vi "Auto Run.vi"() -> ()   [LabVIEW 2016]
uses:
  Ctls/Auto Steps.ctl
  <vilib>/vision/Image Controls.llb/IMAQ Image.ctl
  <vilib>/userdefined/High Color/IMAQdx.ctl
  <vilib>/vision/driver/IMAQdx.llb/IMAQdx Acquisition Mode.ctl
  LCOD.llb/GUI Command.ctl
  <vilib>/vision/driver/IMAQdx.llb/IMAQdx Buffer Number Mode.ctl
  <vilib>/Utility/config.llb/Read Key (Double).vi
  <vilib>/Utility/config.llb/Read Key (String).vi
  <vilib>/vision/driver/NI_Vision_Acquisition_Software.lvlib
  <vilib>/Utility/config.llb/NI_LVConfig.lvlib
panel:
  out "RobSnap":dbl[](array[numeric])
  out "RobRef":dbl[](array[numeric])
  out "CamRef":dbl[](array[numeric])
  out "Calibrate":string caption="值"
  out "Position":sgl[](array[numeric])
  out "Angle":sgl
  out "Top":cluster{"下边缘设置：":i32, "右边缘设置：":i32}
  out "Bottom":cluster{"上边缘设置：":i32, "右边缘设置：":i32}
  # "自动运行函数"
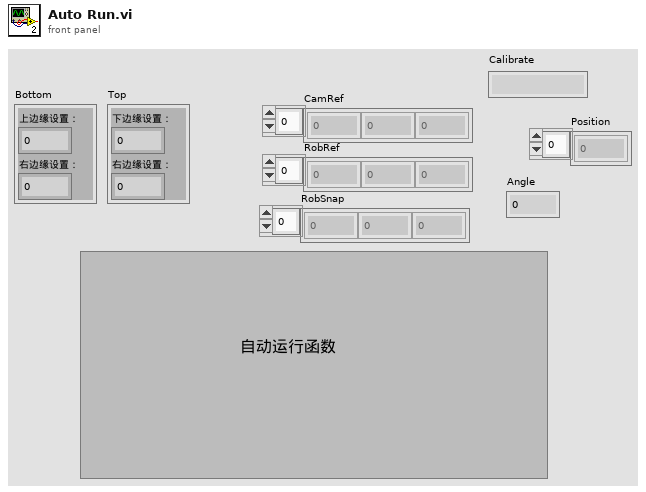
[diagram p1: front panel]
types:
  T1 = typedef "IMAQ Image.ctl" = refnum<image>
  T2 = typedef "Auto Steps.ctl" = enum16{"Nothing", "Initial", "ReadConf", "WaitTrigger", "SnapOnce", "Rotate180", "SnapSecond", "SendPos", "Error", "Pause", "Exit"}
  T3 = typedef "GUI Command.ctl" = enum16{"Under Range", "Get UI Setting", "错误代码处理", "保存数据", "保存图片", "Update Disp_Lists", "Update Sts", "Clear Disp_Lists", "Update Disp_Result", "Clear Disp_Result", "Set Passed Unit", "Set Failed Unit", "Set Total Unit", "Over Range"}
  T4 = typedef "NI_Vision_Acquisition_Software.lvlib/IMAQdx Acquisition Mode.ctl" = enum32{"One Shot", "Continuous"}
  T5 = typedef "IMAQdx.ctl" = refnum<k21>
  T6 = enum16{"Standard", "Buffered", "CRLF", "Immediate"}
  T7 = typedef "NI_Vision_Acquisition_Software.lvlib/IMAQdx Buffer Number Mode.ctl" = enum32{"Next", "Last", "Buffer Number", "Every", "Last New"}
  T8 = typedef "NI_LVConfig.lvlib/Config Data RefNum.ctl" = refnum<k1>
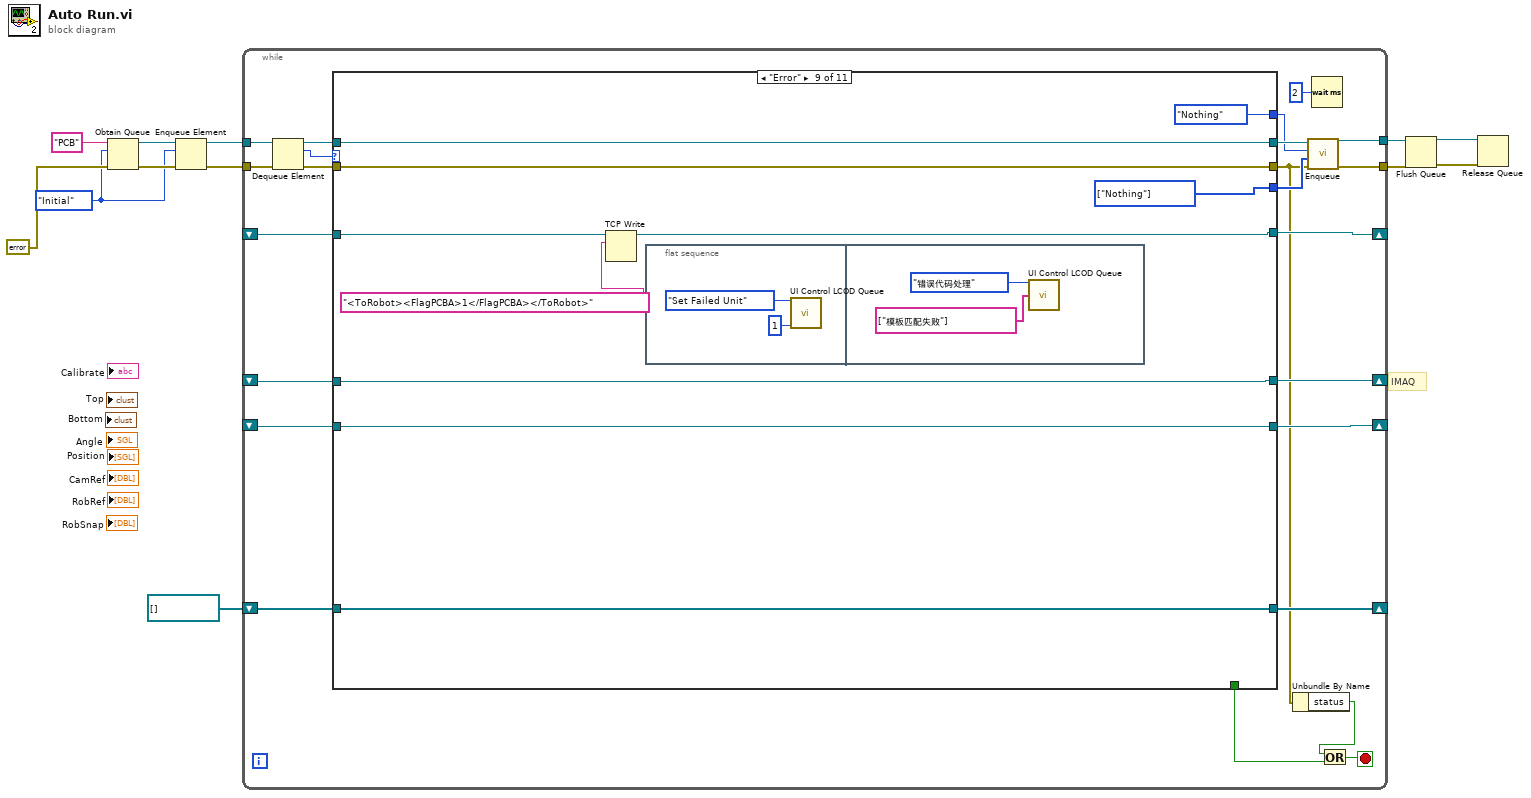
[diagram p0: block diagram]
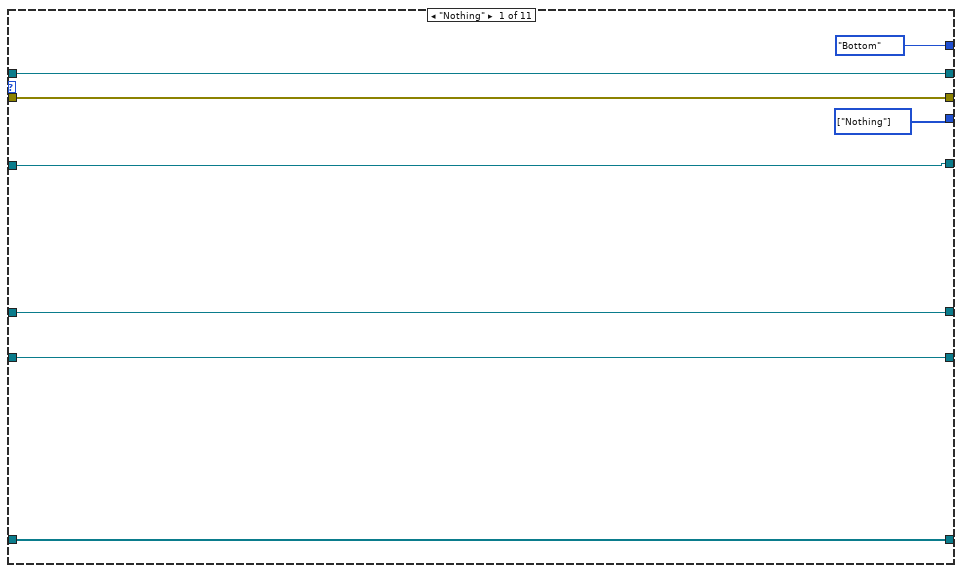
[diagram p2: hidden frame]
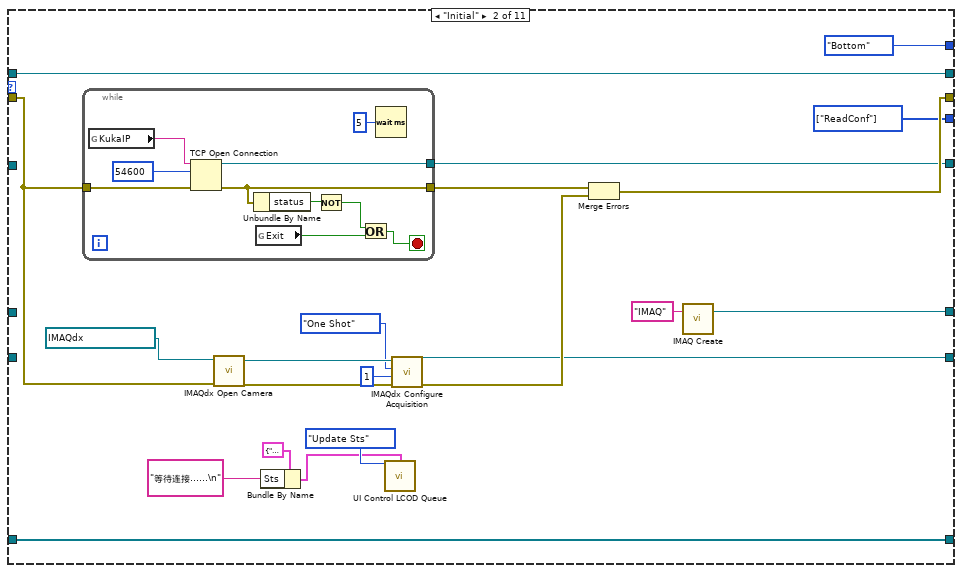
[diagram p3: hidden frame]
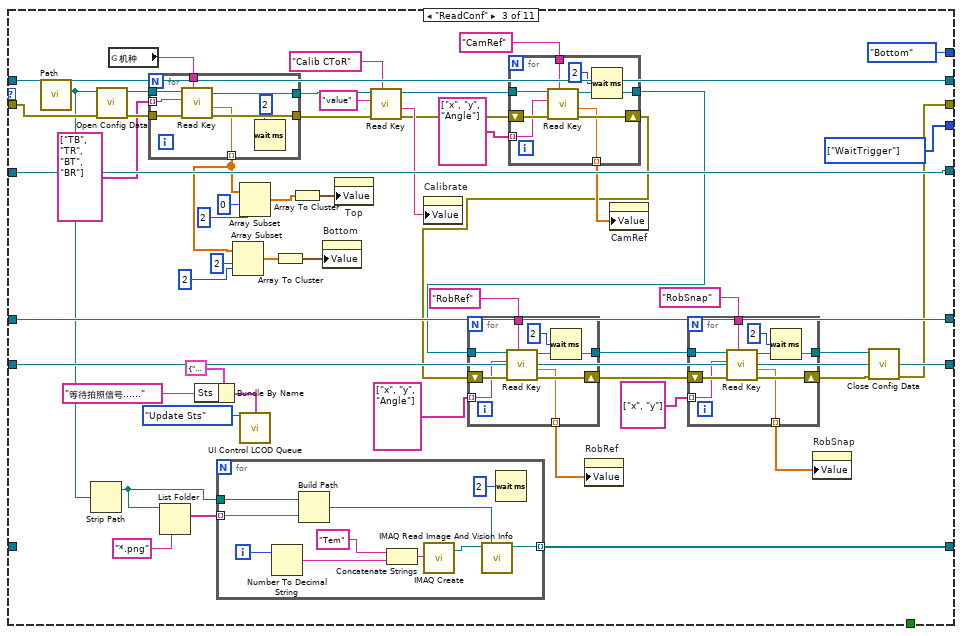
[diagram p4: hidden frame]
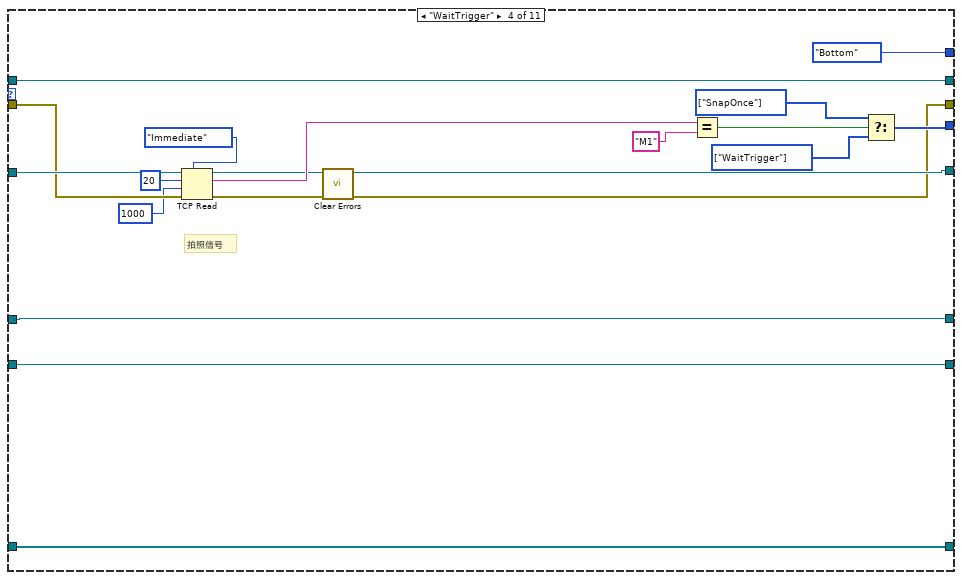
[diagram p5: hidden frame]
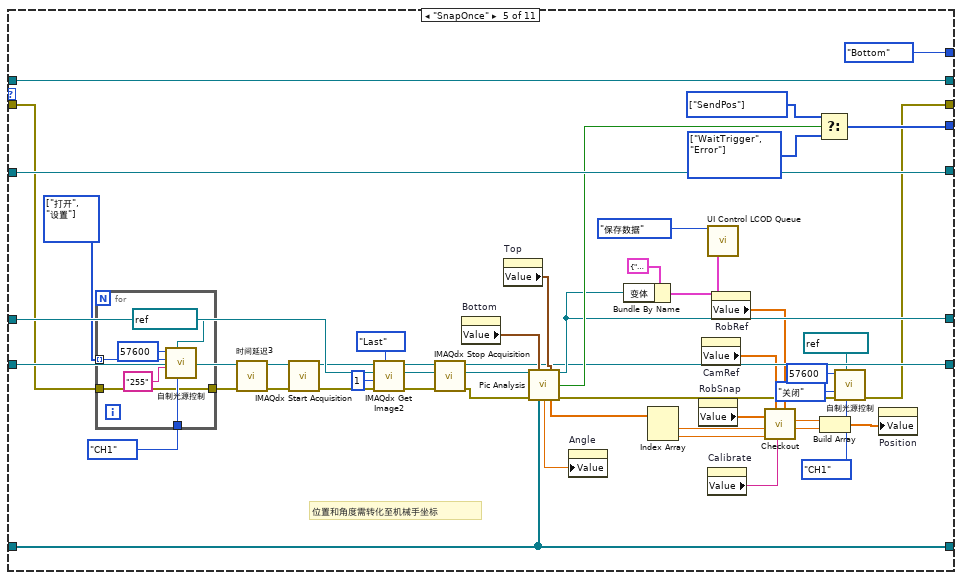
[diagram p6: hidden frame]
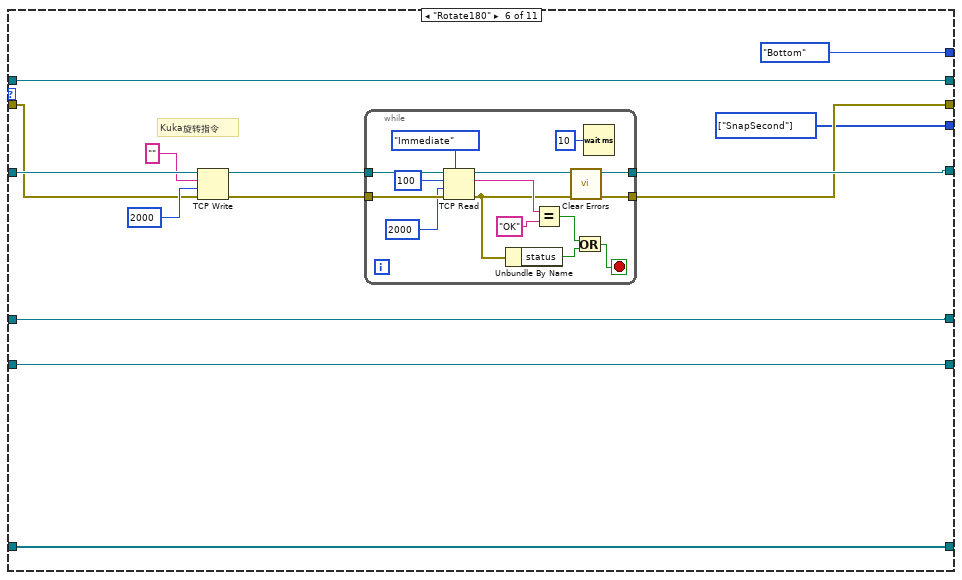
[diagram p7: hidden frame]
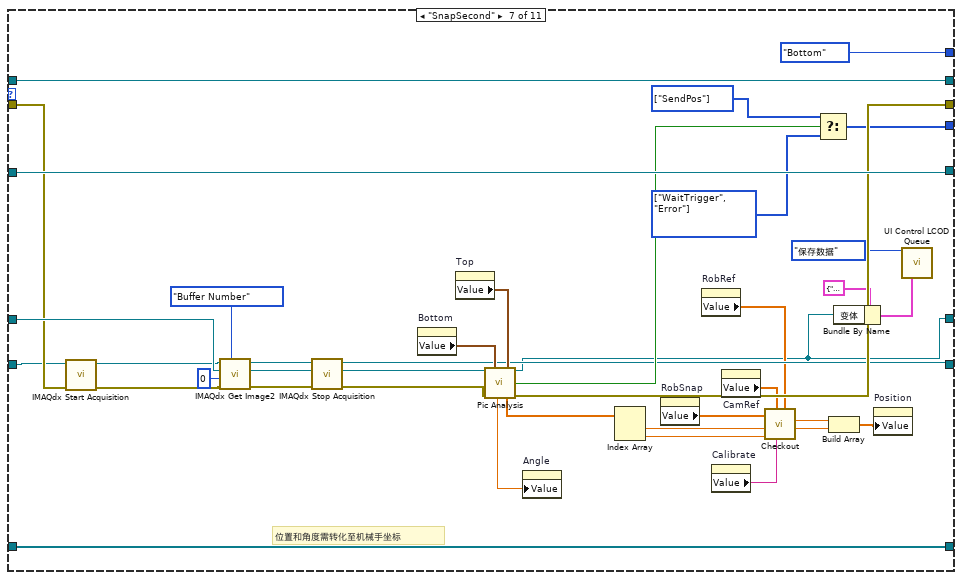
[diagram p8: hidden frame]
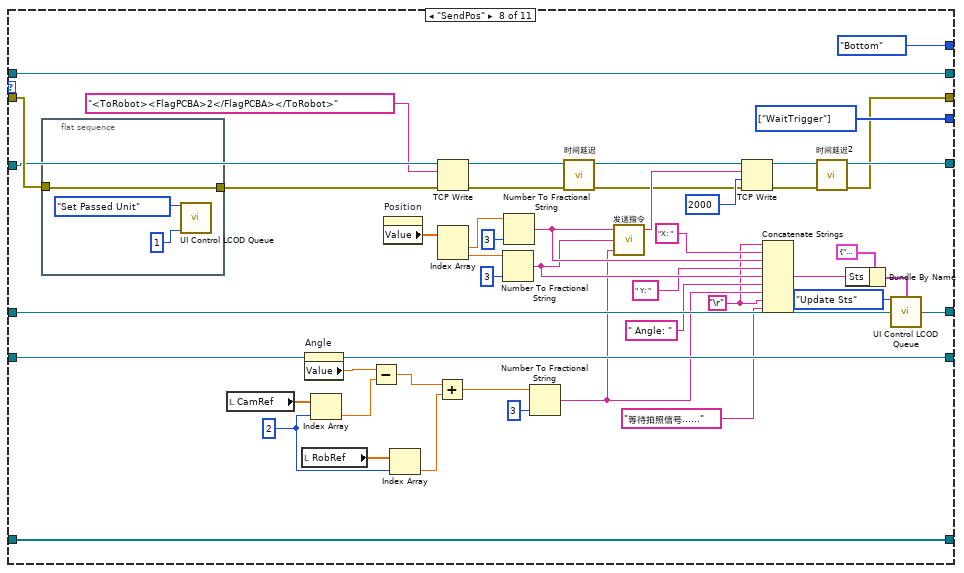
[diagram p9: hidden frame]
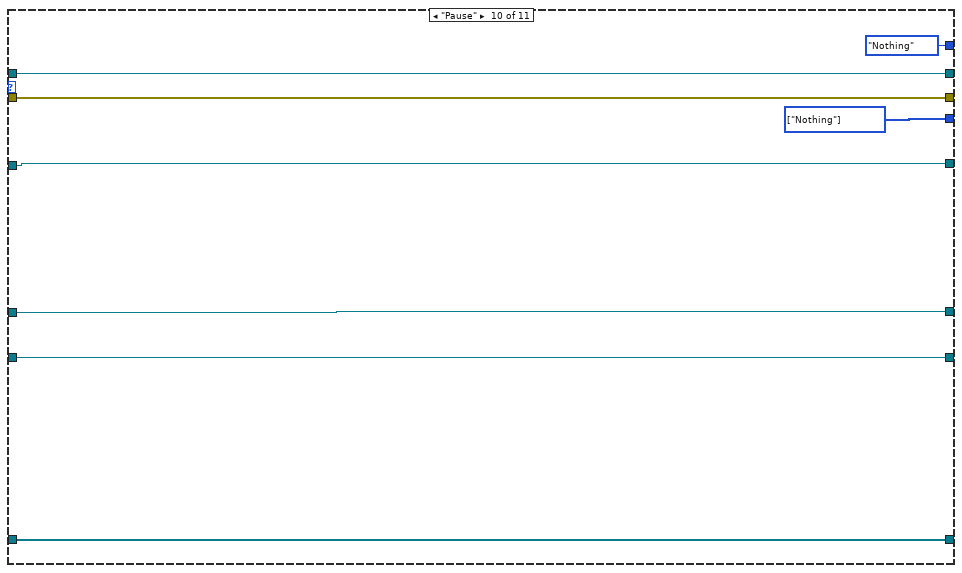
[diagram p10: hidden frame]
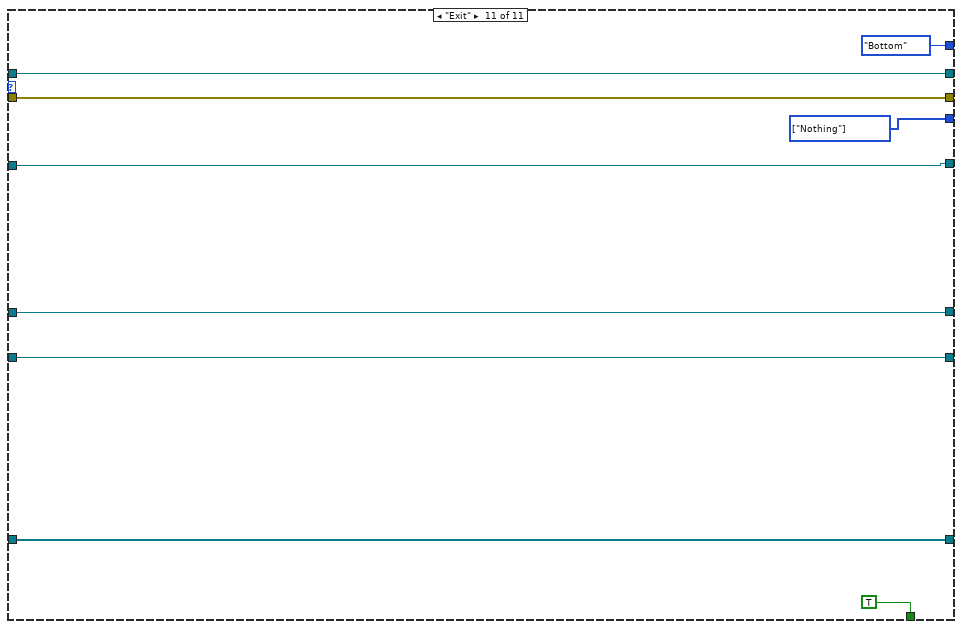
[diagram p11: hidden frame]
diagram:
  w8 = Auto_Steps."Initial"
  # "IMAQ"
  n1 = Obtain Queue(name (unnamed)="PCB" ("名称（未命名）"), element data type=w8, error in (no error)=errorcluster {"status"=FALSE, "code"=0, "source"=""} ("错误输入（无错误）")) -> (queue out=w10:refnum<queue>, error out=w9:errorcluster)  [unwired: 2 in, 1 out]
  n2 = Enqueue Element(queue=w10, element=w8, error in (no error)=w9) -> (queue out=w7:refnum<queue>, error out=w6:errorcluster)  [unwired: 1 in, 1 out]
  n3 = while {
    tunnel: w7 -> [w35]
    tunnel: w6 -> [w34]
    tunnel: [w29] -> w5
    tunnel: [w28] -> w4
    shift-right: [w24] -> _
    shift-left: _ -> [w22]
    shift-right: [w25] -> _
    shift-left: _ -> [w23]
    shift-right: [w21] -> _
    shift-left: _ -> [w20]
    shift-right: [w17] -> _
    shift-left: T1[] [] ("数组") -> [w18]
    stop <- w16 stop-if-true
    n4 = Dequeue Element(queue=w35, error in (no error)=w34) -> (queue out=w32:refnum<queue>, element=w33:T2, error out=w30:errorcluster)  [unwired: 1 in, 1 out]
    n5 = case shown="\"Error\"" w33 {
      tunnel: w32 -> [w43 w64 w126 w187 w234 w254 w306 w350 w363 w375 w383]
      tunnel: [w43 w64 w126 w187 w234 w254 w306 w350 w363 w375 w383] -> w31
      tunnel: w30 -> [w42 w58 w120 w183 w198 w250 w280 w320 w362 w374 w382]
      tunnel: [w42 w53 w118 w171 w193 w246 w297 w310 w362 w374 w382] -> w14
      tunnel: [w37 w51 w101 w179 w226 w242 w296 w331 w358 w369 w377] -> w19
      tunnel: [enum16{"Top", "Bottom", "Nothing"}."Bottom" ("Comd") enum16{"Top", "Bottom", "Nothing"}."Bottom" ("Comd") enum16{"Top", "Bottom", "Nothing"}."Bottom" ("Comd") enum16{"Top", "Bottom", "Nothing"}."Bottom" ("Comd") enum16{"Top", "Bottom", "Nothing"}."Bottom" ("Comd") enum16{"Top", "Bottom", "Nothing"}."Bottom" ("Comd") enum16{"Top", "Bottom", "Nothing"}."Bottom" ("Comd") enum16{"Top", "Bottom", "Nothing"}."Bottom" ("Comd") enum16{"Top", "Bottom", "Nothing"}."Nothing" ("Comd") enum16{"Top", "Bottom", "Nothing"}."Nothing" ("Comd") enum16{"Top", "Bottom", "Nothing"}."Bottom" ("Comd")] -> w26
      tunnel: [w38 w49 w123 w175 w205 w243 w281 w341 w359 w371 w378] -> w25
      tunnel: [w39 w54 w124 w176 w221 w244 w270 w342 w360 w372 w379] -> w24
      tunnel: w23 -> [w38 _ w123 w175 w208 w243 w278 w341 w359 w371 w378]
      tunnel: w22 -> [w39 _ w124 w176 w232 w244 w303 w342 w360 w372 w379]
      tunnel: [w40 w52 w125 w178 w233 w247 w304 w329 w356 w370 w380] -> w21
      tunnel: w20 -> [w40 _ w125 w186 w233 w252 w304 w319 w357 w370 w380]
      tunnel: [_ _ _ _ _ _ _ _ _ _ TRUE] -> w15
      tunnel: w18 -> [w36 w48 _ w169 w188 w241 w269 w307 w354 w368 w376]
      tunnel: [w36 w48 w79 w169 w188 w241 w269 w307 w354 w368 w376] -> w17
      frame "Nothing" {
        w37 = T2[] [enum."Nothing"] items=["Nothing", "Initial", "ReadConf", "WaitTrigger", "SnapOnce", "Rotate180", "SnapSecond", "SendPos", "Error", "Pause", "Exit"]
      }
      frame "Initial" {
        w51 = T2[] [enum."ReadConf"] items=["Nothing", "Initial", "ReadConf", "WaitTrigger", "SnapOnce", "Rotate180", "SnapSecond", "SendPos", "Error", "Pause", "Exit"]
        n6 = while {
          tunnel: [w72] -> w52
          tunnel: w58 -> [w73]
          tunnel: [w70] -> w56
          stop <- w66 stop-if-true
          n7 = global read "全局 1.vi" "KukaIP"() -> (w74:string)
          n8 = TCP Open Connection(address=w74, remote port or service name=u16 54600 ("远程端口或服务名称"), error in (no error)=w73) -> (connection ID=w72:refnum<k5>, error out=w70:errorcluster)  [unwired: 2 in]
          n9 = Unbundle By Name(w70) -> ("status"=w69:bool)
          n10 = global read "全局 1.vi" "Exit"() -> (w67:bool)
          n11 = Not(x=w69) -> (.not. x?=w68:bool)
          n12 = Or(x=w68, y=w67) -> (x .or. y?=w66:bool)
          n13 = Wait (ms)(milliseconds to wait=u32 5 ("等待时间（毫秒）")) -> ()  [unwired: 1 out]
        }
        n14 = call <vilib>:"IMAQdx Open Camera.vi"("error in"=w58, "Session In"=T5 "acA1600-20gc") -> ("error out"=w62:errorcluster, "Session Out"=w61:T5)  [unwired: 8 in]
        n15 = Bundle By Name(cluster=cluster{"工站":string, "Sts":string} {"工站"="", "Sts"=""} ("update Sts In"), "Sts"="等待连接……\n" ("字符串")) -> (w44:cluster{"工站":string, "Sts":string})
        n16 = call "UI Control LCOD Queue.vi"("GUI Command"=GUI_Command."Update Sts", "update Sts In"=w44) -> ()  [unwired: 7 in, 7 out]
        n17 = call <vilib>:"IMAQdx Configure Acquisition.vi"("error in"=w62, "Number of Buffers"=u32 1, "Continuous?"=IMAQdx_Acquisition_Mode."One Shot", "Session In"=w61) -> ("error out"=w50:errorcluster, "Session Out"=w49:T5)  [unwired: 6 in]
        n18 = Merge Errors(w56, w50) -> (w53:errorcluster)
        n19 = call "IMAQ Create"("Image Name"="IMAQ") -> ("New Image"=w54:T1)  [unwired: 4 in, 1 out]
      }
      frame "ReadConf" {
        w101 = T2[] [enum."WaitTrigger"] items=["Nothing", "Initial", "ReadConf", "WaitTrigger", "SnapOnce", "Rotate180", "SnapSecond", "SendPos", "Error", "Pause", "Exit"]
        n20 = call "Path.vi"() -> ("ini"=w83:path)  [unwired: 11 in]
        n21 = Strip Path(path=w83) -> (stripped path=w80:path)  [unwired: 1 out]
        n22 = call <vilib>:"Open Config Data.vi"("error in (no error)"=w120, "configuration file path"=w83) -> ("error out"=w121:errorcluster, "refnum"=w122:T8)  [unwired: 7 in, 1 out]
        n23 = global read "全局 1.vi" "机种"() -> (w119:string)
        n24 = for {
          tunnel: w122 -> [w168]
          tunnel: w121 -> [w167]
          tunnel: w119 -> [w166]
          tunnel: string[] ["TB", "TR", "BT", "BR"] -> [w165] mode=indexing
          tunnel: [w164] -> w107
          tunnel: [w163] -> w106
          tunnel: [w162] -> w102 mode=indexing
          n25 = call-poly <vilib>:"Read Key.vi"("section"=w166, "error in (no error)"=w167, "key"=w165, "refnum"=w168) -> ("error out"=w163:errorcluster, "value"=w162:dbl, "refnum out"=w164:T8)  [unwired: 4 in, 1 out]
          n26 = Wait (ms)(milliseconds to wait=u32 2 ("等待时间（毫秒）")) -> ()  [unwired: 1 out]
        }
        n27 = List Folder(path=w80, pattern="*.png" ("模式")) -> (filenames=w82:string[])  [unwired: 2 in, 3 out]
        n28 = Bundle By Name(cluster=cluster{"工站":string, "Sts":string} {"工站"="", "Sts"=""} ("update Sts In"), "Sts"="等待拍照信号……" ("字符串")) -> (w75:cluster{"工站":string, "Sts":string})
        n29 = for {
          tunnel: w82 -> [w135] mode=indexing
          tunnel: w80 -> [w136]
          tunnel: [w133] -> w79 mode=indexing
          i -> [w129]
          n30 = Number To Decimal String(number=w129) -> (decimal integer string=w128:string)  [unwired: 1 in]
          n31 = Build Path(base path=w136, name or relative path=w135) -> (appended path=w134:path)
          n32 = Concatenate Strings("Tem" ("Image Name"), w128) -> (w132:string)
          n33 = call "IMAQ Create"("Image Name"=w132) -> ("New Image"=w130:T1)  [unwired: 4 in, 1 out]
          n34 = call "IMAQ Read Image And Vision Info"("File Path"=w134, "Image"=w130) -> ("Image Out"=w133:T1)  [unwired: 7 in, 2 out]
          n35 = Wait (ms)(milliseconds to wait=u32 2 ("等待时间（毫秒）")) -> ()  [unwired: 1 out]
        }
        n36 = Array Subset(array=w102, index=2 ("索引"), length=2 ("长度")) -> (w109:dbl[])
        n37 = Array Subset(array=w102, index=0 ("索引"), length=2 ("长度")) -> (w113:dbl[])
        n38 = call "UI Control LCOD Queue.vi"("GUI Command"=GUI_Command."Update Sts", "update Sts In"=w75) -> ()  [unwired: 7 in, 7 out]
        n39 = Array To Cluster(array=w109) -> (cluster=w108:cluster{"[0]":dbl, "[1]":dbl})
        n40 = Array To Cluster(array=w113) -> (cluster=w112:cluster{"[0]":dbl, "[1]":dbl})
        n41 = property on="Bottom" class="Clust (严格)"("Value"=w108) -> ()  [unwired: 2 in, 2 out]
        n42 = property on="Top" class="Clust (严格)"("Value"=w112) -> ()  [unwired: 2 in, 2 out]
        n43 = call-poly <vilib>:"Read Key.vi"("section"="Calib CToR", "error in (no error)"=w106, "key"="value", "refnum"=w107) -> ("error out"=w100:errorcluster, "value"=w103:string, "refnum out"=w99:T8)  [unwired: 4 in, 1 out]
        n44 = property on="Calibrate" class="Str"("Value"=w103) -> ()  [unwired: 2 in, 2 out]
        n45 = for {
          shift-right: [w159] -> w95
          shift-left: w100 -> [w160]
          tunnel: w99 -> [w158]
          tunnel: [w157] -> w92
          tunnel: string[] ["x", "y", "Angle"] -> [w156] mode=indexing
          tunnel: "CamRef" ("key") -> [w155]
          tunnel: [w153] -> w96 mode=indexing
          n46 = call-poly <vilib>:"Read Key.vi"("section"=w155, "error in (no error)"=w160, "key"=w156, "refnum"=w158) -> ("error out"=w159:errorcluster, "value"=w153:dbl, "refnum out"=w157:T8)  [unwired: 4 in, 1 out]
          n47 = Wait (ms)(milliseconds to wait=u32 2 ("等待时间（毫秒）")) -> ()  [unwired: 1 out]
        }
        n48 = for {
          shift-right: [w151] -> w89
          shift-left: w95 -> [w152]
          tunnel: w92 -> [w150]
          tunnel: [w149] -> w90
          tunnel: string[] ["x", "y", "Angle"] -> [w148] mode=indexing
          tunnel: "RobRef" ("key") -> [w147]
          tunnel: [w145] -> w91 mode=indexing
          n49 = call-poly <vilib>:"Read Key.vi"("section"=w147, "error in (no error)"=w152, "key"=w148, "refnum"=w150) -> ("error out"=w151:errorcluster, "value"=w145:dbl, "refnum out"=w149:T8)  [unwired: 4 in, 1 out]
          n50 = Wait (ms)(milliseconds to wait=u32 2 ("等待时间（毫秒）")) -> ()  [unwired: 1 out]
        }
        n51 = property on="RobRef" class="Arr (严格)"("Value"=w91) -> ()  [unwired: 2 in, 2 out]
        n52 = property on="CamRef" class="Arr (严格)"("Value"=w96) -> ()  [unwired: 2 in, 2 out]
        n53 = for {
          shift-right: [w143] -> w84
          shift-left: w89 -> [w144]
          tunnel: w90 -> [w142]
          tunnel: [w141] -> w85
          tunnel: string[] ["x", "y"] -> [w140] mode=indexing
          tunnel: "RobSnap" ("key") -> [w139]
          tunnel: [w137] -> w86 mode=indexing
          n54 = call-poly <vilib>:"Read Key.vi"("section"=w139, "error in (no error)"=w144, "key"=w140, "refnum"=w142) -> ("error out"=w143:errorcluster, "value"=w137:dbl, "refnum out"=w141:T8)  [unwired: 4 in, 1 out]
          n55 = Wait (ms)(milliseconds to wait=u32 2 ("等待时间（毫秒）")) -> ()  [unwired: 1 out]
        }
        n56 = property on="RobSnap" class="Arr (严格)"("Value"=w86) -> ()  [unwired: 2 in, 2 out]
        n57 = call <vilib>:"Close Config Data.vi"("error in (no error)"=w84, "refnum"=w85) -> ("error out"=w118:errorcluster)  [unwired: 8 in, 1 out]
      }
      frame "WaitTrigger" {
        w173 = T2[] [enum."WaitTrigger"] items=["Nothing", "Initial", "ReadConf", "WaitTrigger", "SnapOnce", "Rotate180", "SnapSecond", "SendPos", "Error", "Pause", "Exit"]
        w174 = T2[] [enum."SnapOnce"] items=["Nothing", "Initial", "ReadConf", "WaitTrigger", "SnapOnce", "Rotate180", "SnapSecond", "SendPos", "Error", "Pause", "Exit"]
        # "拍照信号"
        n58 = TCP Read(connection ID=w186, bytes to read=20 ("读取的字节"), error in (no error)=w183, 7:T6."Immediate" ("模式（标准）"), 9:1000 ("超时毫秒(25000)")) -> (connection ID out=w178:refnum<k5>, data out=w182:string, error out=w172:errorcluster)
        n59 = call <vilib>:"Clear Errors.vi"("error in (no error)"=w172) -> ("error out"=w171:errorcluster)  [unwired: 5 in, 1 out]
        n60 = Equal?(x=w182, y="M1") -> (x = y?=w180:bool)
        n61 = Select(t=w174, s=w180, f=w173) -> (s? t:f=w179:T2[])
      }
      frame "SnapOnce" {
        w197 = enum16{"打开", "关闭", "设置"}[] [enum."打开", enum."设置"] items=["打开", "关闭", "设置"]
        w210 = T2[] [enum."WaitTrigger", enum."Error"] items=["Nothing", "Initial", "ReadConf", "WaitTrigger", "SnapOnce", "Rotate180", "SnapSecond", "SendPos", "Error", "Pause", "Exit"]
        w211 = T2[] [enum."SendPos"] items=["Nothing", "Initial", "ReadConf", "WaitTrigger", "SnapOnce", "Rotate180", "SnapSecond", "SendPos", "Error", "Pause", "Exit"]
        # "位置和角度需转化至机械手坐标"
        n62 = for {
          tunnel: enum16{"CH1", "CH2", "CH3", "CH4"}."CH1" ("通道") -> [w237]
          tunnel: [w236] -> w196
          tunnel: w198 -> [w236]
          tunnel: w197 -> [w235] mode=indexing
          n63 = call "自制光源控制.vi"("通道"=w237, "VISA In"=refnum<visa-resource-name> "COM1", "亮度"="255", "操作模式"=w235, "baud rate"=u32 57600) -> ()  [unwired: 4 in, 3 out]
        }
        n64 = call "时间延迟3"("error in (no error)"=w196) -> ("error out"=w195:errorcluster)  [unwired: 10 in]
        n65 = call <vilib>:"IMAQdx Start Acquisition.vi"("error in"=w195, "Session In"=w208) -> ("error out"=w209:errorcluster, "Session Out"=w207:T5)  [unwired: 8 in]
        n66 = call <vilib>:"IMAQdx Get Image2.vi"("Buffer Number Mode (Next)"=IMAQdx_Buffer_Number_Mode."Last", "error in"=w209, "Buffer Number In"=u32 1, "Image In"=w232, "Session In"=w207) -> ("error out"=w204:errorcluster, "Image Out"=w228:T1, "Session Out"=w206:T5)  [unwired: 3 in, 1 out]
        n67 = call <vilib>:"IMAQdx Stop Acquisition.vi"("error in"=w204, "Session In"=w206) -> ("error out"=w203:errorcluster, "Session Out"=w205:T5)  [unwired: 8 in]
        n68 = property on="Bottom" class="Clust (严格)"() -> ("Value"=w229:cluster{"上边缘设置：":i32, "右边缘设置：":i32})  [unwired: 2 in, 2 out]
        n69 = property on="Top" class="Clust (严格)"() -> ("Value"=w230:cluster{"下边缘设置：":i32, "右边缘设置：":i32})  [unwired: 2 in, 2 out]
        n70 = call "Pic Analysis.vi"("Image in"=w228, "Bottom"=w229, "Top"=w230, "error in"=w203, "Temp"=w188) -> ("Image"=w221:T1, "Found"=w225:bool, "Angle"=w227:sgl, "Position"=w218:sgl[], "错误输出"=w194:errorcluster)  [unwired: 5 in, 1 out]
        n71 = property on="Angle" class="DigNum (严格)"("Value"=w227) -> ()  [unwired: 2 in, 2 out]
        n72 = Bundle By Name(cluster=cluster{"String":string, "变体":variant} {"String"="", "变体"=variant} ("保存图片输入"), "变体"=w221) -> (w220:cluster{"String":string, "变体":variant})
        n73 = Index Array(array=w218) -> (element #1=w217:sgl, element #2=w216:sgl)  [unwired: 2 in]
        n74 = property on="RobSnap" class="Arr (严格)"() -> ("Value"=w200:dbl[])  [unwired: 2 in, 2 out]
        n75 = property on="CamRef" class="Arr (严格)"() -> ("Value"=w202:dbl[])  [unwired: 2 in, 2 out]
        n76 = call "UI Control LCOD Queue.vi"("GUI Command"=GUI_Command."保存数据", "保存图片输入"=w220) -> ()  [unwired: 7 in, 7 out]
        n77 = property on="Calibrate" class="Str"() -> ("Value"=w215:string)  [unwired: 2 in, 2 out]
        n78 = property on="RobRef" class="Arr (严格)"() -> ("Value"=w201:dbl[])  [unwired: 2 in, 2 out]
        n79 = call "Checkout.vi"("RobRef"=w201, "Array"=w215, "CamRef"=w202, "camera y"=w216, "camera x"=w217, "RobSnap"=w200) -> ("robot y"=w213:dbl, "robot x"=w214:dbl)  [unwired: 4 in]
        n80 = Select(t=w211, s=w225, f=w210) -> (s? t:f=w226:T2[])
        n81 = Build Array(w214, w213) -> (w212:dbl[])
        n82 = call "自制光源控制.vi"("通道"=enum16{"CH1", "CH2", "CH3", "CH4"}."CH1", "VISA In"=refnum<visa-resource-name> "COM1", "错误输入"=w194, "操作模式"=enum16{"打开", "关闭", "设置"}."关闭", "baud rate"=u32 57600) -> ("错误输出"=w193:errorcluster)  [unwired: 4 in, 2 out]
        n83 = property on="Position" class="Arr (严格)"("Value"=w212) -> ()  [unwired: 2 in, 2 out]
      }
      frame "Rotate180" {
        w242 = T2[] [enum."SnapSecond"] items=["Nothing", "Initial", "ReadConf", "WaitTrigger", "SnapOnce", "Rotate180", "SnapSecond", "SendPos", "Error", "Pause", "Exit"]
        # "Kuka旋转指令"
        n84 = TCP Write(connection ID=w252, data in="" ("数据输入"), error in (no error)=w250, 9:2000 ("超时毫秒(25000)")) -> (connection ID out=w249:refnum<k5>, error out=w248:errorcluster)  [unwired: 1 out]
        n85 = while {
          tunnel: w249 -> [w268]
          tunnel: w248 -> [w267]
          tunnel: [w258] -> w247
          tunnel: [w255] -> w246
          stop <- w261 stop-if-true
          n86 = TCP Read(connection ID=w268, bytes to read=100 ("读取的字节"), error in (no error)=w267, 7:T6."Immediate" ("模式（标准）"), 9:2000 ("超时毫秒(25000)")) -> (connection ID out=w258:refnum<k5>, data out=w263:string, error out=w256:errorcluster)
          n87 = Unbundle By Name(w256) -> ("status"=w259:bool)
          n88 = Equal?(x=w263, y="OK") -> (x = y?=w260:bool)
          n89 = call <vilib>:"Clear Errors.vi"("error in (no error)"=w256) -> ("error out"=w255:errorcluster)  [unwired: 5 in, 1 out]
          n90 = Or(x=w260, y=w259) -> (x .or. y?=w261:bool)
          n91 = Wait (ms)(milliseconds to wait=u32 10 ("等待时间（毫秒）")) -> ()  [unwired: 1 out]
        }
      }
      frame "SnapSecond" {
        w285 = T2[] [enum."SendPos"] items=["Nothing", "Initial", "ReadConf", "WaitTrigger", "SnapOnce", "Rotate180", "SnapSecond", "SendPos", "Error", "Pause", "Exit"]
        w286 = T2[] [enum."WaitTrigger", enum."Error"] items=["Nothing", "Initial", "ReadConf", "WaitTrigger", "SnapOnce", "Rotate180", "SnapSecond", "SendPos", "Error", "Pause", "Exit"]
        # "位置和角度需转化至机械手坐标"
        n92 = call <vilib>:"IMAQdx Start Acquisition.vi"("error in"=w280, "Session In"=w278) -> ("error out"=w279:errorcluster, "Session Out"=w277:T5)  [unwired: 8 in]
        n93 = call <vilib>:"IMAQdx Get Image2.vi"("Buffer Number Mode (Next)"=IMAQdx_Buffer_Number_Mode."Buffer Number", "error in"=w279, "Buffer Number In"=u32 0, "Image In"=w303, "Session In"=w277) -> ("error out"=w284:errorcluster, "Image Out"=w301:T1, "Session Out"=w282:T5)  [unwired: 3 in, 1 out]
        n94 = call <vilib>:"IMAQdx Stop Acquisition.vi"("error in"=w284, "Session In"=w282) -> ("error out"=w283:errorcluster, "Session Out"=w281:T5)  [unwired: 8 in]
        n95 = property on="Bottom" class="Clust (严格)"() -> ("Value"=w298:cluster{"上边缘设置：":i32, "右边缘设置：":i32})  [unwired: 2 in, 2 out]
        n96 = property on="Top" class="Clust (严格)"() -> ("Value"=w299:cluster{"下边缘设置：":i32, "右边缘设置：":i32})  [unwired: 2 in, 2 out]
        n97 = call "Pic Analysis.vi"("Image in"=w301, "Bottom"=w298, "Top"=w299, "error in"=w283) -> ("Image"=w270:T1, "Found"=w295:bool, "Angle"=w300:sgl, "Position"=w294:sgl[], "错误输出"=w297:errorcluster)  [unwired: 6 in, 1 out]
        n98 = property on="Angle" class="DigNum (严格)"("Value"=w300) -> ()  [unwired: 2 in, 2 out]
        n99 = Index Array(array=w294) -> (element #1=w293:sgl, element #2=w292:sgl)  [unwired: 2 in]
        n100 = property on="RobSnap" class="Arr (严格)"() -> ("Value"=w274:dbl[])  [unwired: 2 in, 2 out]
        n101 = property on="RobRef" class="Arr (严格)"() -> ("Value"=w275:dbl[])  [unwired: 2 in, 2 out]
        n102 = property on="Calibrate" class="Str"() -> ("Value"=w291:string)  [unwired: 2 in, 2 out]
        n103 = property on="CamRef" class="Arr (严格)"() -> ("Value"=w276:dbl[])  [unwired: 2 in, 2 out]
        n104 = call "Checkout.vi"("RobRef"=w275, "Array"=w291, "CamRef"=w276, "camera y"=w292, "camera x"=w293, "RobSnap"=w274) -> ("robot y"=w289:dbl, "robot x"=w290:dbl)  [unwired: 4 in]
        n105 = Select(t=w285, s=w295, f=w286) -> (s? t:f=w296:T2[])
        n106 = Build Array(w290, w289) -> (w288:dbl[])
        n107 = Bundle By Name(cluster=cluster{"String":string, "变体":variant} {"String"="", "变体"=variant} ("保存图片输入"), "变体"=w270) -> (w271:cluster{"String":string, "变体":variant})
        n108 = property on="Position" class="Arr (严格)"("Value"=w288) -> ()  [unwired: 2 in, 2 out]
        n109 = call "UI Control LCOD Queue.vi"("GUI Command"=GUI_Command."保存数据", "保存图片输入"=w271) -> ()  [unwired: 7 in, 7 out]
      }
      frame "SendPos" {
        w308 = "\r"
        w321 = 2 ("索引")
        w331 = T2[] [enum."WaitTrigger"] items=["Nothing", "Initial", "ReadConf", "WaitTrigger", "SnapOnce", "Rotate180", "SnapSecond", "SendPos", "Error", "Pause", "Exit"]
        n110 = flat-sequence {
          tunnel: w320 -> [w351]
          tunnel: [w351] -> w317
          frame #0 {
            n111 = call "UI Control LCOD Queue.vi"("GUI Command"=GUI_Command."Set Passed Unit", "Count"=1) -> ()  [unwired: 7 in, 7 out]
          }
        }
        n112 = local read "CamRef"() -> (w328:dbl[])
        n113 = local read "RobRef"() -> (w326:dbl[])
        n114 = property on="Angle" class="DigNum (严格)"() -> ("Value"=w327:sgl)  [unwired: 2 in, 2 out]
        n115 = Index Array(array=w328, index=w321) -> (element=w323:dbl)
        n116 = Subtract(x=w327, y=w323) -> (x-y=w325:dbl)
        n117 = property on="Position" class="Arr (严格)"() -> ("Value"=w349:sgl[])  [unwired: 2 in, 2 out]
        n118 = Index Array(array=w326, index=w321) -> (element=w322:dbl)
        n119 = Add(x=w325, y=w322) -> (x+y=w324:dbl)
        n120 = TCP Write(connection ID=w319, data in="<ToRobot><FlagPCBA>2</FlagPCBA></ToRobot>" ("数据输入"), error in (no error)=w317) -> (connection ID out=w318:refnum<k5>, error out=w313:errorcluster)  [unwired: 1 in, 1 out]
        n121 = Index Array(array=w349) -> (element #1=w348:sgl, element #2=w345:sgl)  [unwired: 2 in]
        n122 = Number To Fractional String(number=w345, precision (6)=i16 3 ("精度(6)")) -> (F-format string=w337:string)  [unwired: 2 in]
        n123 = Number To Fractional String(number=w348, precision (6)=i16 3 ("精度(6)")) -> (F-format string=w338:string)  [unwired: 2 in]
        n124 = Number To Fractional String(number=w324, precision (6)=i16 3 ("精度(6)")) -> (F-format string=w330:string)  [unwired: 2 in]
        n125 = call "时间延迟"("error in (no error)"=w313) -> ("error out"=w312:errorcluster)  [unwired: 10 in]
        n126 = call "发送指令.vi"("C"=w330, "Y"=w337, "X"=w338) -> ("发送指令"=w344:string)  [unwired: 2 in]
        n127 = TCP Write(connection ID=w318, data in=w344, error in (no error)=w312, 9:2000 ("超时毫秒(25000)")) -> (connection ID out=w329:refnum<k5>, error out=w311:errorcluster)  [unwired: 1 out]
        n128 = Concatenate Strings(w308, "X: " ("字符串"), w338, " Y: ", w337, " Angle: ", w330, w308, "等待拍照信号……" ("字符串")) -> (w333:string)
        n129 = call "时间延迟2"("error in (no error)"=w311) -> ("error out"=w310:errorcluster)  [unwired: 10 in]
        n130 = Bundle By Name(cluster=cluster{"工站":string, "Sts":string} {"工站"="", "Sts"=""} ("update Sts In"), "Sts"=w333) -> (w332:cluster{"工站":string, "Sts":string})
        n131 = call "UI Control LCOD Queue.vi"("GUI Command"=GUI_Command."Update Sts", "update Sts In"=w332) -> ()  [unwired: 7 in, 7 out]
      }
      frame "Error" {
        w358 = T2[] [enum."Nothing"] items=["Nothing", "Initial", "ReadConf", "WaitTrigger", "SnapOnce", "Rotate180", "SnapSecond", "SendPos", "Error", "Pause", "Exit"]
        n132 = TCP Write(connection ID=w357, data in="<ToRobot><FlagPCBA>1</FlagPCBA></ToRobot>" ("数据输入")) -> (connection ID out=w356:refnum<k5>)  [unwired: 2 in, 2 out]
        n133 = flat-sequence {
          frame #0 {
            n134 = call "UI Control LCOD Queue.vi"("GUI Command"=GUI_Command."Set Failed Unit", "Count"=1) -> ()  [unwired: 7 in, 7 out]
          }
          frame #1 {
            n135 = call "UI Control LCOD Queue.vi"("GUI Command"=GUI_Command."错误代码处理", "错误代码输入"=string[] ["模板匹配失败"]) -> ()  [unwired: 7 in, 7 out]
          }
        }
      }
      frame "Pause" {
        w369 = T2[] [enum."Nothing"] items=["Nothing", "Initial", "ReadConf", "WaitTrigger", "SnapOnce", "Rotate180", "SnapSecond", "SendPos", "Error", "Pause", "Exit"]
      }
      frame "Exit" {
        w377 = T2[] [enum."Nothing"] items=["Nothing", "Initial", "ReadConf", "WaitTrigger", "SnapOnce", "Rotate180", "SnapSecond", "SendPos", "Error", "Pause", "Exit"]
      }
    }
    n136 = Unbundle By Name(w14) -> ("status"=w13:bool)
    n137 = call "Enqueue.vi"("错误输入（无错误）"=w14, "Steps"=w19, "Comd"=w26, "队列输入"=w31) -> ("error out"=w28:errorcluster, "队列输出"=w29:refnum<queue>)  [unwired: 6 in]
    n138 = Wait (ms)(milliseconds to wait=u32 2 ("等待时间（毫秒）")) -> ()  [unwired: 1 out]
    n139 = Or(x=w13, y=w15) -> (x .or. y?=w16:bool)
  }
  n140 = Flush Queue(queue=w5, error in (no error)=w4) -> (queue out=w3:refnum<queue>, error out=w2:errorcluster)  [unwired: 1 out]
  n141 = Release Queue(queue=w3, error in (no error)=w2) -> ()  [unwired: 1 in, 3 out]
